vi "PercentDifference.vi"(2 "Basis":dbl, 3 "Comparee":dbl) -> (1 "PercentageDifference":dbl)   [LabVIEW 2012]
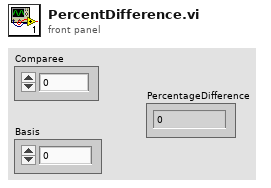
[diagram p1: front panel]
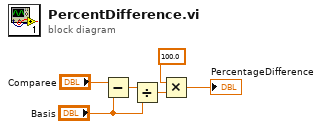
[diagram p0: block diagram]
diagram:
  n1 = Subtract(x="Comparee", y="Basis") -> (x-y=w1:dbl)
  n2 = Divide(x=w1, y="Basis") -> (x/y=w2:dbl)
  n3 = Multiply(x=100.0 ("y"), y=w2) -> (x*y=→"PercentageDifference":dbl)
